vi "Write wavelength.vi"(8 "error in (no error)":errorcluster, 10 "wavelength":T1=400.0, 11 "ChangeWavelength in":refnum<class "ChangeWavelength.lvclass">) -> (0 "error out":errorcluster, 3 "ChangeWavelength out":refnum<class "ChangeWavelength.lvclass">)   [LabVIEW 2020, in "ChangeWavelength.lvclass"]
uses:
  ChangeWavelength.lvclass
  Typedefs/wavelength.ctl
  ChangeWavelength.lvclass/ChangeWavelength.ctl
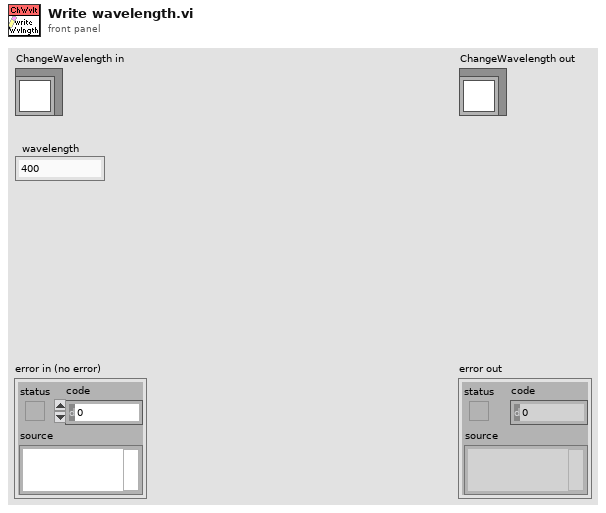
[diagram p1: front panel]
types:
  T1 = typedef "wavelength.ctl" = dbl
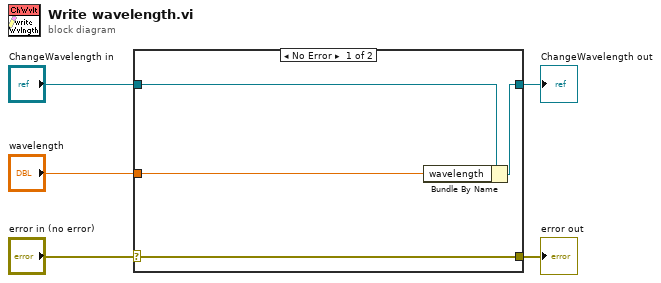
[diagram p0: block diagram]
diagram:
  n1 = case shown="No Error" "error in (no error)" {
    selector: "error in (no error)" -> [w9 w10]
    tunnel: [w9 w10] -> w4
    tunnel: [w7 w11] -> w2
    tunnel: "ChangeWavelength in" -> [w8 w11]
    tunnel: "wavelength" -> [w6 _]
    frame No Error {
      n2 = Bundle By Name(cluster=w8, "wavelength"=w6) -> (w7:refnum<class "ChangeWavelength.lvclass">)
    }
    frame Error {
    }
  }
  "error out" <- w4
  "ChangeWavelength out" <- w2
